vi "Automatic CE-CERT Inverter MODBUS TCP-IP Power Factor.vi"() -> ()   [LabVIEW 2018]
uses:
  <vilib>/Plasmionique/MB Master/MB_Master_TCP/MB_Master_TCP.lvclass
  C:/Program Files (x86)/National Instruments/LabVIEW 2018/vi.lib/Plasmionique/MB Master/MB_Master/MB_Master.lvclass
  <vilib>/Plasmionique/MB Master/MB Master.lvlib
panel:
  in  "power factor":u16
  out "Power Factor Format Error (0)":u16
  out "3035 Register Value":u16
  out "Power Factor Mode Read Back (Step 10)":u16
  out "Power Factor Operation Error (Step 9)(Can Read 0 or 10)":u16
  out "Power Factor Operation Error (Step 1)(Should Read 0)":u16
  in  "IP Address":string
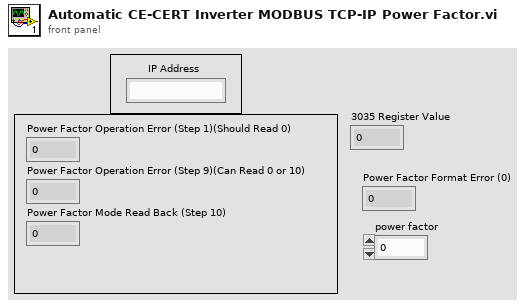
[diagram p1: front panel]
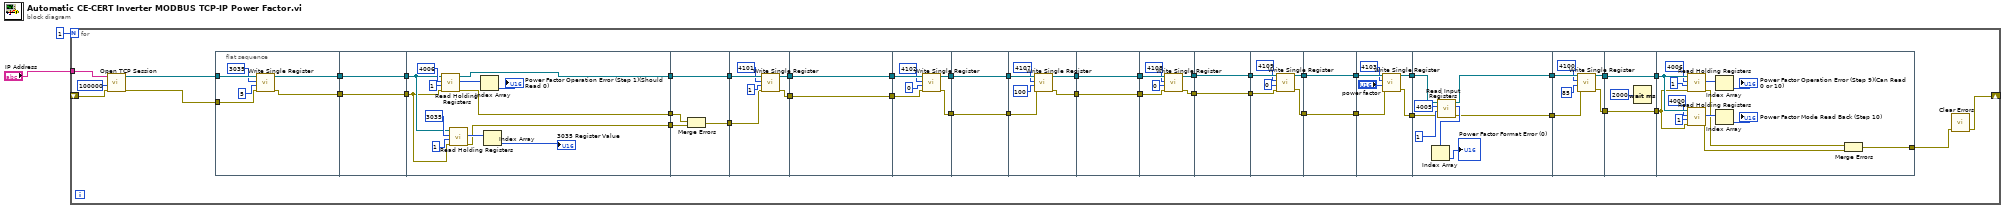
[diagram p0: block diagram]
diagram:
  n1 = for {
    N: 1 -> [_]
    tunnel: "IP Address" -> [w28]
    shift-right: [w4] -> _
    shift-left: _ -> [w25]
    n2 = call <vilib>:"Open TCP Session.vi"("error in (no error)"=w25, "Timeout (10000)"=100000, "IP Address"=w28) -> ("error out"=w24:errorcluster, "MB_TCP session"=w27:refnum<class "MB_Master_TCP.lvclass">)  [unwired: 7 in]
    n3 = flat-sequence {
      tunnel: w27 -> [w52]
      tunnel: [w49] -> w29
      tunnel: w24 -> [w48]
      tunnel: [w47] -> w22
      tunnel: [w54] -> w30
      tunnel: w29 -> [w54]
      tunnel: [w53] -> w23
      tunnel: w22 -> [w53]
      tunnel: [w65] -> w46
      tunnel: w30 -> [w60]
      tunnel: w23 -> [w57]
      tunnel: [w56] -> w21
      tunnel: [w55] -> w20
      tunnel: w46 -> [w71]
      tunnel: [w71] -> w45
      tunnel: w21 -> [w70]
      tunnel: w20 -> [w69]
      tunnel: [w68] -> w19
      tunnel: w45 -> [w77]
      tunnel: [w74] -> w44
      tunnel: w19 -> [w73]
      tunnel: [w72] -> w17
      tunnel: w44 -> [w79]
      tunnel: [w79] -> w43
      tunnel: [w78] -> w18
      tunnel: w17 -> [w78]
      tunnel: w43 -> [w85]
      tunnel: [w82] -> w42
      tunnel: w18 -> [w81]
      tunnel: [w80] -> w15
      tunnel: w42 -> [w87]
      tunnel: [w87] -> w41
      tunnel: [w86] -> w16
      tunnel: w15 -> [w86]
      tunnel: w41 -> [w93]
      tunnel: [w92] -> w40
      tunnel: w16 -> [w89]
      tunnel: [w88] -> w13
      tunnel: w40 -> [w95]
      tunnel: [w95] -> w39
      tunnel: [w94] -> w14
      tunnel: w13 -> [w94]
      tunnel: w39 -> [w101]
      tunnel: [w98] -> w38
      tunnel: w14 -> [w97]
      tunnel: [w96] -> w11
      tunnel: w38 -> [w103]
      tunnel: [w103] -> w37
      tunnel: [w102] -> w12
      tunnel: w11 -> [w102]
      tunnel: w37 -> [w109]
      tunnel: [w106] -> w36
      tunnel: w12 -> [w105]
      tunnel: [w104] -> w9
      tunnel: w36 -> [w111]
      tunnel: [w111] -> w35
      tunnel: [w110] -> w10
      tunnel: w9 -> [w110]
      tunnel: w35 -> [w117]
      tunnel: [w115] -> w34
      tunnel: w10 -> [w114]
      tunnel: [w113] -> w8
      tunnel: w34 -> [w125]
      tunnel: [w124] -> w33
      tunnel: w8 -> [w119]
      tunnel: [w118] -> w7
      tunnel: w33 -> [w131]
      tunnel: [w128] -> w32
      tunnel: w7 -> [w127]
      tunnel: [w126] -> w5
      tunnel: w32 -> [w134]
      tunnel: [w134] -> w31
      tunnel: [w132] -> w6
      tunnel: w5 -> [w132]
      tunnel: w31 -> [w147]
      tunnel: w6 -> [w138]
      tunnel: [w135] -> w3
      frame #0 {
        n4 = call <vilib>:"Write Single Register.vi"("error in (no error)"=w48, "value"=u16 5, "address"=u16 3035, "MB session in"=w52) -> ("error out"=w47:errorcluster, "MB session out"=w49:refnum<class "MB_Master_TCP.lvclass">)  [unwired: 6 in]
      }
      frame #1 {
      }
      frame #2 {
        n5 = call <vilib>:"Read Holding Registers.vi"("error in (no error)"=w57, "quantity"=u16 1, "starting address"=u16 4006, "MB session in"=w60) -> ("error out"=w55:errorcluster, "Registers"=w67:u16[], "MB session out"=w65:refnum<class "MB_Master_TCP.lvclass">)  [unwired: 5 in]
        n6 = call <vilib>:"Read Holding Registers.vi"("error in (no error)"=w57, "quantity"=u16 1, "starting address"=u16 3035, "MB session in"=w60) -> ("error out"=w56:errorcluster, "Registers"=w59:u16[])  [unwired: 5 in, 1 out]
        n7 = Index Array(array=w67) -> (element=→"Power Factor Operation Error (Step 1)(Should Read 0)":u16)  [unwired: 1 in]
        n8 = Index Array(array=w59) -> (element=→"3035 Register Value":u16)  [unwired: 1 in]
      }
      frame #3 {
        n9 = Merge Errors(w69, w70) -> (w68:errorcluster)
      }
      frame #4 {
        n10 = call <vilib>:"Write Single Register.vi"("error in (no error)"=w73, "value"=u16 1, "address"=u16 4101, "MB session in"=w77) -> ("error out"=w72:errorcluster, "MB session out"=w74:refnum<class "MB_Master_TCP.lvclass">)  [unwired: 6 in]
      }
      frame #5 {
      }
      frame #6 {
        n11 = call <vilib>:"Write Single Register.vi"("error in (no error)"=w81, "value"=u16 0, "address"=u16 4102, "MB session in"=w85) -> ("error out"=w80:errorcluster, "MB session out"=w82:refnum<class "MB_Master_TCP.lvclass">)  [unwired: 6 in]
      }
      frame #7 {
      }
      frame #8 {
        n12 = call <vilib>:"Write Single Register.vi"("error in (no error)"=w89, "value"=u16 100, "address"=u16 4107, "MB session in"=w93) -> ("error out"=w88:errorcluster, "MB session out"=w92:refnum<class "MB_Master_TCP.lvclass">)  [unwired: 6 in]
      }
      frame #9 {
      }
      frame #10 {
        n13 = call <vilib>:"Write Single Register.vi"("error in (no error)"=w97, "value"=u16 0, "address"=u16 4108, "MB session in"=w101) -> ("error out"=w96:errorcluster, "MB session out"=w98:refnum<class "MB_Master_TCP.lvclass">)  [unwired: 6 in]
      }
      frame #11 {
      }
      frame #12 {
        n14 = call <vilib>:"Write Single Register.vi"("error in (no error)"=w105, "value"=u16 0, "address"=u16 4109, "MB session in"=w109) -> ("error out"=w104:errorcluster, "MB session out"=w106:refnum<class "MB_Master_TCP.lvclass">)  [unwired: 6 in]
      }
      frame #13 {
      }
      frame #14 {
        n15 = call <vilib>:"Write Single Register.vi"("error in (no error)"=w114, "value"="power factor", "address"=u16 4103, "MB session in"=w117) -> ("error out"=w113:errorcluster, "MB session out"=w115:refnum<class "MB_Master_TCP.lvclass">)  [unwired: 6 in]
      }
      frame #15 {
        n16 = call <vilib>:"Read Input Registers.vi"("error in (no error)"=w119, "quantity"=u16 1, "starting address"=u16 4005, "MB session in"=w125) -> ("error out"=w118:errorcluster, "Registers"=w121:u16[], "MB session out"=w124:refnum<class "MB_Master_TCP.lvclass">)  [unwired: 5 in]
        n17 = Index Array(array=w121) -> (element=→"Power Factor Format Error (0)":u16)  [unwired: 1 in]
      }
      frame #16 {
        n18 = call <vilib>:"Write Single Register.vi"("error in (no error)"=w127, "value"=u16 85, "address"=u16 4100, "MB session in"=w131) -> ("error out"=w126:errorcluster, "MB session out"=w128:refnum<class "MB_Master_TCP.lvclass">)  [unwired: 6 in]
      }
      frame #17 {
        n19 = Wait (ms)(milliseconds to wait=u32 2000) -> ()  [unwired: 1 out]
      }
      frame #18 {
        n20 = call <vilib>:"Read Holding Registers.vi"("error in (no error)"=w138, "quantity"=u16 1, "starting address"=u16 4006, "MB session in"=w147) -> ("error out"=w137:errorcluster, "Registers"=w142:u16[])  [unwired: 5 in, 1 out]
        n21 = call <vilib>:"Read Holding Registers.vi"("error in (no error)"=w138, "quantity"=u16 1, "starting address"=u16 4000, "MB session in"=w147) -> ("error out"=w136:errorcluster, "Registers"=w141:u16[])  [unwired: 5 in, 1 out]
        n22 = Index Array(array=w142) -> (element=→"Power Factor Operation Error (Step 9)(Can Read 0 or 10)":u16)  [unwired: 1 in]
        n23 = Index Array(array=w141) -> (element=→"Power Factor Mode Read Back (Step 10)":u16)  [unwired: 1 in]
        n24 = Merge Errors(w137, w136) -> (w135:errorcluster)
      }
    }
    n25 = call <vilib>:"Clear Errors.vi"("error in (no error)"=w3) -> ("error out"=w4:errorcluster)  [unwired: 5 in, 1 out]
  }
